vi "1717-2_CommandDemo.vi"() -> ()   [LabVIEW 2012, in "Lib_UEL.ATE.lvlib" / "Lib_IPVoice.lvlib"]
uses:
  Lib_IPVoice.lvlib
panel:
  in  "Value":u8[](array[numeric])
  out "错误输出 2":errorcluster={"status"=TRUE, "code"=56, "source"="TCP Listen.vi:1->1717-2_CommandDemo.vi中的等待TCP侦听器"} caption="错误输出"
  out "连接的字符串":string
  out "数据输出":string
  out "Data_Out":u8[](array[numeric])=[1] format="%02x"
  out "OP_Status":i16=1
  in  "Register":T1(ring)=enum."debugmode"
  out "错误输出":errorcluster
  in  "Command":enum16{"Connect", "Read", "Write", "DisConnect"}(ring)=enum."Read"
  in  "停止":bool
  in  "RUN":bool
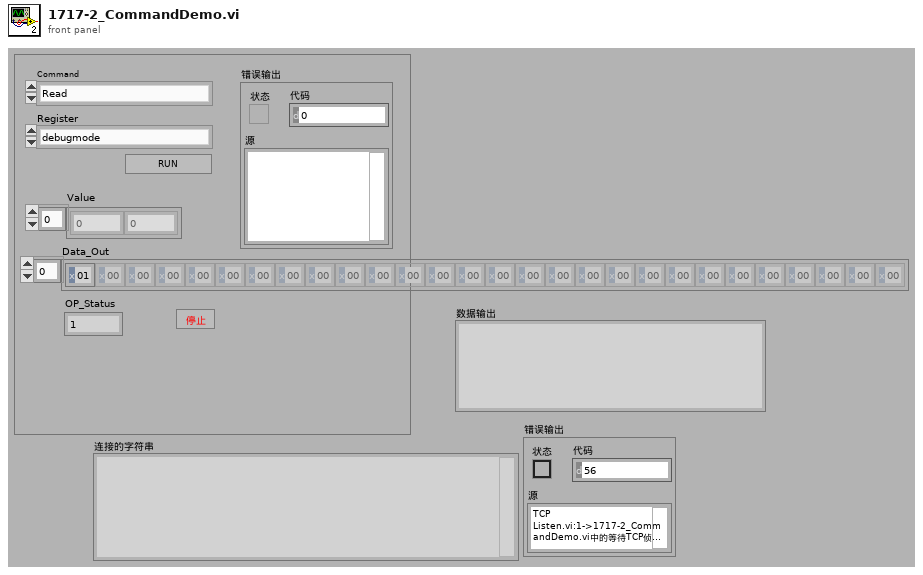
[diagram p1: front panel]
types:
  T1 = enum16{"Device_Type", "FWVersion", "debugmode", "sw_upgr_avail", "dbg_serial", "dbg_touch", "dbg_touch_x", "dbg_touch_y", "dbg_sd_status", "dbg_sd_write", "dbg_sd_write_res", "dbg_bright", "dbg_usb", "dbg_usb_res", "dbg_usb_sc", "dbg_ila", "dbg_hs", "dbg_hs_push", "dbg_hs_rec", "dbg_hs_rec_res", "dbg_hs_play", "dbg_led_mute", "dbg_led_allarm", "dbg_led_message", "dbg_led_door", "dbg_led_logo", "dbg_led_logo1", "dbg_aux_ring", "dbg_floor_call", "dbg_panic", "dbg_soft_on", "dbg_wifi", "dbg_wifi_res", "dbg_calibr_status", "dbg_calibr_status_res", "dbg_delta_cal", "dbg_calibrate", "dbg_calibrate_res", "dbg_audioin", "dbg_audioin_res", "dbg_audioin_offset", "dbg_audioout_left", "dbg_audioout_left_offset", "dbg_audioout_right", "dbg_audioout_right_offset", "dbg_audioout_6dB", "dbg_display", "dbg_video_loopback", "dbg_mac1", "dbg_mac2", "dbg_mac_wifi", "dbg_mac_bt", "dbg_mac_zigbee", "dbg_touch_aux", "dbg_audioout_mono", "dbg_touch_out"}
  T2 = enum16{"Standard", "Buffered", "CRLF", "Immediate"}
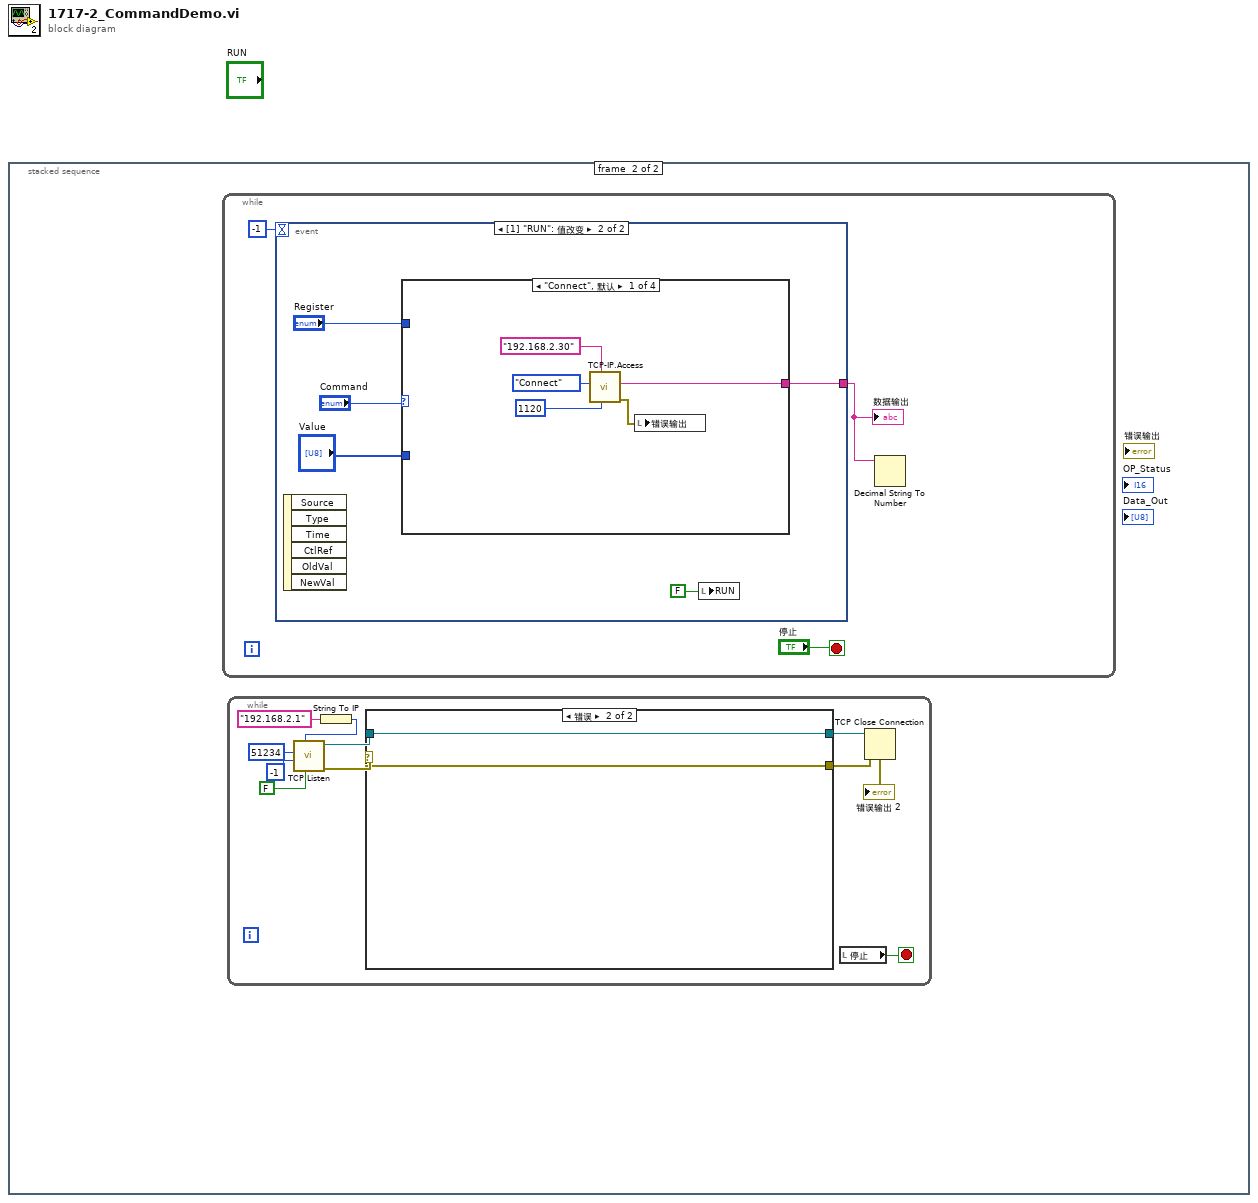
[diagram p0: block diagram]
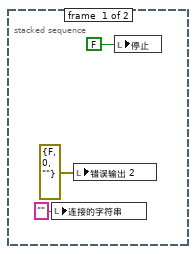
[diagram p2: hidden frame]
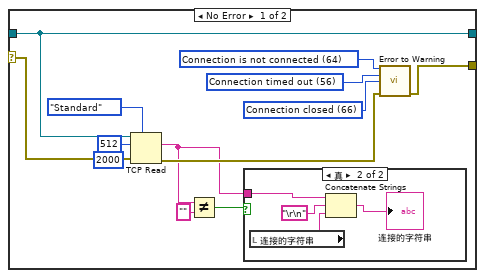
[diagram p3: hidden frame]
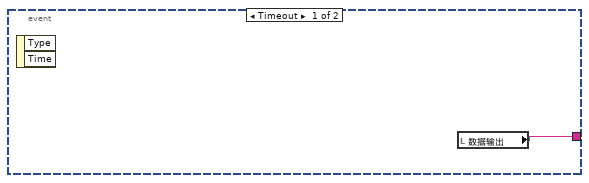
[diagram p5: hidden frame]
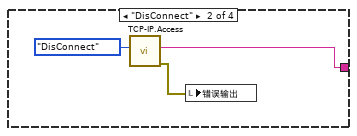
[diagram p6: hidden frame]
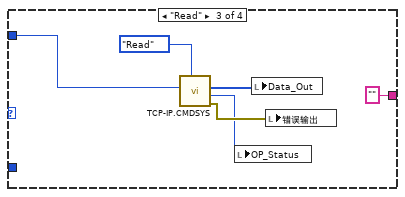
[diagram p7: hidden frame]
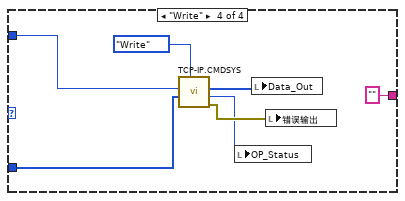
[diagram p8: hidden frame]
diagram:
  n1 = stacked-sequence {
    frame #0 {
      n2 = local write "连接的字符串"("" ("连接的字符串")) -> ()
      n3 = local write "错误输出 2"(errorcluster {"status"=FALSE, "code"=0, "source"=""} ("错误输出 2")) -> ()
      n4 = local write "停止"(FALSE ("停止")) -> ()
    }
    frame #1 {
      n5 = while {
        stop <- "停止" stop-if-true
        n6 = event shown="[1] \"RUN\": 值改变" {
          selector: _ -> [_ _]
          dyn-events: _ -> [_ _]
          timeout: -1 -> [_ _]
          tunnel: [w37 w42] -> w35
          event Timeout {
            n7 = event-data() -> ()  [unwired: 1 in, 2 out]
            n8 = local read "数据输出"() -> (w37:string)
          }
          event "RUN": Value Change {
            n9 = event-data() -> ()  [unwired: 1 in, 6 out]
            n10 = case shown="\"Connect\", 默认" "Command" {
              tunnel: "Register" -> [_ _ w55 w62]
              tunnel: "Value" -> [_ _ _ w57]
              tunnel: [w44 w48 "" ("数据输出") "" ("数据输出")] -> w42
              frame "Connect", Default {
                n11 = call "TCP-IP.Access.vi"("本地基端口"=u16 1120, "IP Address"="192.168.2.30", "Command"=enum16{"Connect", "Read", "Write", "DisConnect"}."Connect") -> ("错误输出"=w45:errorcluster, "数据输出"=w44:string)  [unwired: 5 in, 2 out]
                n12 = local write "错误输出"(w45) -> ()
              }
              frame "DisConnect" {
                n13 = call "TCP-IP.Access.vi"("Command"=enum16{"Connect", "Read", "Write", "DisConnect"}."DisConnect") -> ("错误输出"=w50:errorcluster, "数据输出"=w48:string)  [unwired: 7 in, 2 out]
                n14 = local write "错误输出"(w50) -> ()
              }
              frame "Read" {
                n15 = call "TCP-IP.CMDSYS.vi"("Cmd"=enum16{"Read", "Write"}."Read", "Register"=w55) -> ("错误输出"=w54:errorcluster, "OP_Status"=w53:i16, "Data_Out"=w52:u8[])  [unwired: 6 in, 1 out]
                n16 = local write "OP_Status"(w53) -> ()
                n17 = local write "Data_Out"(w52) -> ()
                n18 = local write "错误输出"(w54) -> ()
              }
              frame "Write" {
                n19 = call "TCP-IP.CMDSYS.vi"("Cmd"=enum16{"Read", "Write"}."Write", "Value"=w57, "Register"=w62) -> ("错误输出"=w61:errorcluster, "OP_Status"=w60:i16, "Data_Out"=w59:u8[])  [unwired: 5 in, 1 out]
                n20 = local write "OP_Status"(w60) -> ()
                n21 = local write "Data_Out"(w59) -> ()
                n22 = local write "错误输出"(w61) -> ()
              }
            }
            n23 = local write "RUN"(FALSE ("RUN")) -> ()
          }
        }
        "数据输出" <- w35
        n24 = Decimal String To Number(string=w35) -> ()  [unwired: 2 in, 2 out]
      }
      n25 = while {
        stop <- w7 stop-if-true
        n26 = String To IP(1:"192.168.2.1" ("名称")) -> (0:w14:u32)
        n27 = call <vilib>:"TCP Listen.vi"("resolve remote address (T)"=FALSE, "net address"=w14, "timeout ms (wait forever: -1)"=-1, "port"=u16 51234) -> ("error out"=w11:errorcluster, "connection ID"=w12:refnum<k5>)  [unwired: 3 in, 3 out]
        n28 = case shown="错误" w11 {
          selector: w11 -> [w26 w32]
          tunnel: [w22 w32] -> w8
          tunnel: w12 -> [w27 w33]
          tunnel: [w27 w33] -> w9
          frame No Error {
            w24 = 56 items=["No Error", "Argument Error", "Memory Full", "Out of Zone", "End of File", "File Already Open", "Generic File IO Error", "File Not Found", "File Permission Error", "Disk Full", "Duplicate Path", "Too Many Files Open", "Not Enabled", "Resource File Not Found", "Cannot Add Resource", "Resource Not Found", "Image Not Found", "Image Memory Error", "Pen Does Not Exist", "Config Bad Type", "Config Token Not Found", "Config Parse Error", "Config Memory Error", "Bad External Code Format", "Bad External Code Offset", "External Code Not Present", "Null Window", "Destroy Window Mixup", "Null Menu", "Print Aborted", "Bad Print Record", "Print Driver Error", "Windows Error During Print", "Memory Error During Print", "Print Dialog Error", "Generic Print Error", "Invalid Device Refnum", "Device Not Found", "Device Parameter Error", "Device Unit Error", "Can't Open Device", "Device Call Aborted", "Generic Error", "Cancelled By User", "Object ID Too Low", "Object ID Too High", "Object Not In Heap", "Unknown Heap", "Bad DefProc ID", "DefProc Not In Table", "Message Out Of Range", "Null Method", "Unknown Message", "Manager Call Not Supported", "Bad address", "Connection In progress", "Connection timed out", "Connection is already in progress", "Network attribute not supported", "Network error", "Address in use", "System out of memory", "Connection aborted", "Connection refused", "Connection is not connected", "Connection is already connected", "Connection closed", "Initialize error (interapplication manager)", "Bad occurrence", "Wait on unbound occurrence handler", "Occurrence queue overflow", "Bad path", "Semaphore not signaled", "Unrecognized type (interapplication manager)"] ("2nd Error to Convert")
            w25 = 66 items=["No Error", "Argument Error", "Memory Full", "Out of Zone", "End of File", "File Already Open", "Generic File IO Error", "File Not Found", "File Permission Error", "Disk Full", "Duplicate Path", "Too Many Files Open", "Not Enabled", "Resource File Not Found", "Cannot Add Resource", "Resource Not Found", "Image Not Found", "Image Memory Error", "Pen Does Not Exist", "Config Bad Type", "Config Token Not Found", "Config Parse Error", "Config Memory Error", "Bad External Code Format", "Bad External Code Offset", "External Code Not Present", "Null Window", "Destroy Window Mixup", "Null Menu", "Print Aborted", "Bad Print Record", "Print Driver Error", "Windows Error During Print", "Memory Error During Print", "Print Dialog Error", "Generic Print Error", "Invalid Device Refnum", "Device Not Found", "Device Parameter Error", "Device Unit Error", "Can't Open Device", "Device Call Aborted", "Generic Error", "Cancelled By User", "Object ID Too Low", "Object ID Too High", "Object Not In Heap", "Unknown Heap", "Bad DefProc ID", "DefProc Not In Table", "Message Out Of Range", "Null Method", "Unknown Message", "Manager Call Not Supported", "Bad address", "Connection In progress", "Connection timed out", "Connection is already in progress", "Network attribute not supported", "Network error", "Address in use", "System out of memory", "Connection aborted", "Connection refused", "Connection is not connected", "Connection is already connected", "Connection closed", "Initialize error (interapplication manager)", "Bad occurrence", "Wait on unbound occurrence handler", "Occurrence queue overflow", "Bad path", "Semaphore not signaled", "Unrecognized type (interapplication manager)"] ("3rd Error to Convert")
            w18 = 64 items=["No Error", "Argument Error", "Memory Full", "Out of Zone", "End of File", "File Already Open", "Generic File IO Error", "File Not Found", "File Permission Error", "Disk Full", "Duplicate Path", "Too Many Files Open", "Not Enabled", "Resource File Not Found", "Cannot Add Resource", "Resource Not Found", "Image Not Found", "Image Memory Error", "Pen Does Not Exist", "Config Bad Type", "Config Token Not Found", "Config Parse Error", "Config Memory Error", "Bad External Code Format", "Bad External Code Offset", "External Code Not Present", "Null Window", "Destroy Window Mixup", "Null Menu", "Print Aborted", "Bad Print Record", "Print Driver Error", "Windows Error During Print", "Memory Error During Print", "Print Dialog Error", "Generic Print Error", "Invalid Device Refnum", "Device Not Found", "Device Parameter Error", "Device Unit Error", "Can't Open Device", "Device Call Aborted", "Generic Error", "Cancelled By User", "Object ID Too Low", "Object ID Too High", "Object Not In Heap", "Unknown Heap", "Bad DefProc ID", "DefProc Not In Table", "Message Out Of Range", "Null Method", "Unknown Message", "Manager Call Not Supported", "Bad address", "Connection In progress", "Connection timed out", "Connection is already in progress", "Network attribute not supported", "Network error", "Address in use", "System out of memory", "Connection aborted", "Connection refused", "Connection is not connected", "Connection is already connected", "Connection closed", "Initialize error (interapplication manager)", "Bad occurrence", "Wait on unbound occurrence handler", "Occurrence queue overflow", "Bad path", "Semaphore not signaled", "Unrecognized type (interapplication manager)"] ("1st Error to Convert")
            n29 = TCP Read(connection ID=w27, bytes to read=512 ("读取的字节"), error in (no error)=w26, 7:T2."Standard" ("模式（标准）"), 9:2000 ("超时毫秒(25000)")) -> (data out=w21:string, error out=w23:errorcluster)  [unwired: 1 out]
            n30 = Not Equal?(x=w21, y="") -> (x != y?=w19:bool)
            n31 = case shown="真" w19 {
              tunnel: w21 -> [_ w28]
              frame False {
              }
              frame True {
                n32 = local read "连接的字符串"() -> (w30:string)
                n33 = Concatenate Strings(w28, "\r\n", w30) -> (→"连接的字符串":string)
              }
            }
            n34 = call <vilib>:"Error to Warning.vi"("1st Error to Convert"=w18, "2nd Error to Convert"=w24, "3rd Error to Convert"=w25, "error in"=w23) -> ("warning out"=w22:errorcluster)  [unwired: 11 in]
          }
          frame Error {
          }
        }
        n35 = local read "停止"() -> (w7:bool)
        n36 = TCP Close Connection(connection ID=w9, error in (no error)=w8) -> (error out=→"错误输出 2":errorcluster)  [unwired: 1 in, 1 out]
      }
    }
  }
